vi "Simple Tester.vi"(6 "Action":enum16{"Start Session", "Stop Session"}(ring)) -> ()   [LabVIEW 2020]
doc: "Simple Tester to Start/Stop flexlogger session"
uses:
  FlexLogger_gRPC.lvclass
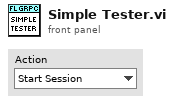
[diagram p1: front panel]
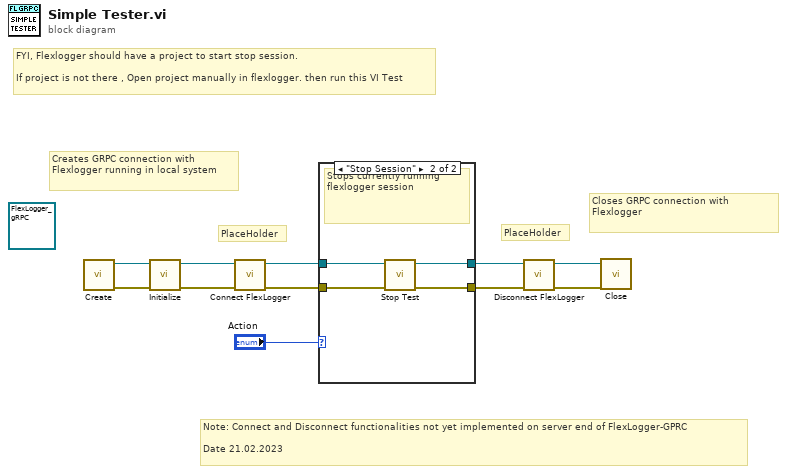
[diagram p0: block diagram]
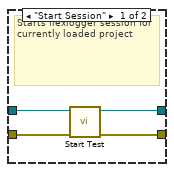
[diagram p2: hidden frame]
diagram:
  (unwired) refnum<class "FlexLogger_gRPC.lvclass"> refnum ("FlexLogger_gRPC.lvlib:FlexLogger_gRPC.lvclass")
  # "FYI, Flexlogger should have a project to start stop session.\n\nIf project is not there , Open project manually in flexlogger. then run this VI Test"
  # "Closes GRPC connection with Flexlogger"
  # "Creates GRPC connection with Flexlogger running in local system"
  # "Note: Connect and Disconnect functionalities not yet implemented on server end of FlexLogger-GPRC \n\nDate 21.02.2023"
  # "PlaceHolder"
  # "PlaceHolder"
  n1 = call "Create.vi"() -> ("error out"=w1:errorcluster, "FlexLogger_gRPC out"=w2:refnum<class "FlexLogger_gRPC.lvclass">)  [unwired: 10 in]
  n2 = call-dynamic "Initialize.vi"("error in (no error)"=w1, "FlexLogger_gRPCAPI in"=w2) -> ("error out"=w10:errorcluster, "FlexLogger_gRPCAPI out"=w11:refnum<class "FlexLogger_gRPC.lvclass">)  [unwired: 8 in]
  n3 = call-dynamic "Connect FlexLogger.vi"("error in (no error)"=w10, "FlexLogger_gRPCAPI in"=w11) -> ("error out"=w8:errorcluster, "FlexLogger_gRPCAPI out"=w9:refnum<class "FlexLogger_gRPC.lvclass">)  [unwired: 8 in]
  n4 = case shown="\"Stop Session\"" "Action" {
    tunnel: w9 -> [w15 w19]
    tunnel: w8 -> [w14 w17]
    tunnel: [w13 w18] -> w7
    tunnel: [w12 w16] -> w5
    frame "Start Session" {
      # "Starts flexlogger session for currently loaded project"
      n5 = call-dynamic "Start Test.vi"("error in (no error)"=w14, "FlexLogger_gRPCAPI in"=w15) -> ("error out"=w12:errorcluster, "FlexLogger_gRPCAPI out"=w13:refnum<class "FlexLogger_gRPC.lvclass">)  [unwired: 7 in, 1 out]
    }
    frame "Stop Session" {
      # "Stops currently running flexlogger session"
      n6 = call-dynamic "Stop Test.vi"("error in (no error)"=w17, "FlexLogger_gRPCAPI in"=w19) -> ("error out"=w16:errorcluster, "FlexLogger_gRPCAPI out"=w18:refnum<class "FlexLogger_gRPC.lvclass">)  [unwired: 8 in]
    }
  }
  n7 = call-dynamic "Disconnect FlexLogger.vi"("error in (no error)"=w5, "FlexLogger_gRPCAPI in"=w7) -> ("error out"=w4:errorcluster, "FlexLogger_gRPCAPI out"=w6:refnum<class "FlexLogger_gRPC.lvclass">)  [unwired: 8 in]
  n8 = call-dynamic "Close.vi"("error in (no error)"=w4, "FlexLogger_gRPC in"=w6) -> ()  [unwired: 8 in, 2 out]
